vi "New JSON ({Boolean[]}).vi"(7 "keys":string[](array[string]), 8 "error in (no error)":errorcluster, 10 "values":bool[](array[boolean])) -> (0 "error out":errorcluster, 3 "JSON Value out":refnum<class "JSON Value.lvclass">)   [LabVIEW 2016, in "JSON Value.lvclass"]
doc: "Create a new JSON Object initialized with the given key value pairs. The key and value arrays must be the same size."
uses:
  JSON Value.lvclass
  Object/Insert Value/Insert Value (Value[]).vi
  New JSON (Boolean).vi
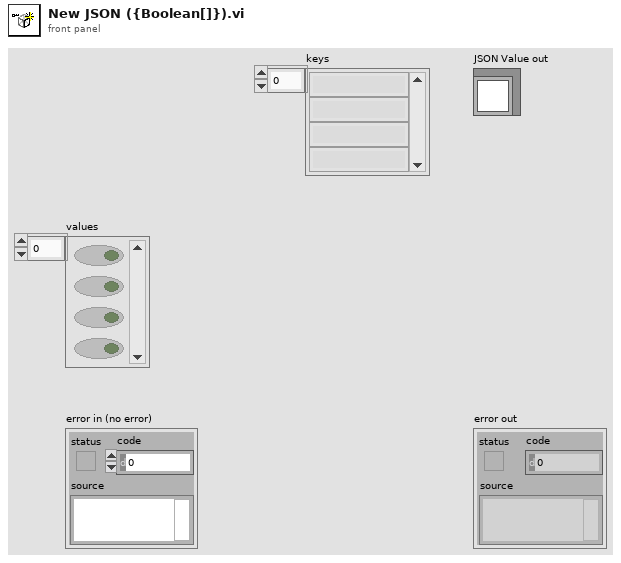
[diagram p1: front panel]
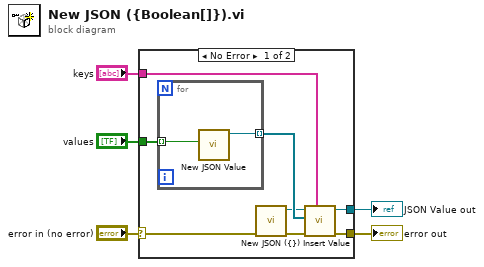
[diagram p0: block diagram]
diagram:
  n1 = case shown="No Error" "error in (no error)" {
    selector: "error in (no error)" -> [w13 w16]
    tunnel: [w12 w16] -> w4
    tunnel: [w11 _] -> w3
    tunnel: "keys" -> [w10 _]
    tunnel: "values" -> [w9 _]
    frame No Error {
      n2 = for {
        tunnel: w9 -> [w15] mode=indexing
        tunnel: [w14] -> w8 mode=indexing
        n3 = call-poly "New JSON Value.vi"("value"=w15) -> ("JSON Value out"=w14:refnum<class "JSON Value.lvclass">)  [unwired: 9 in, 1 out]
      }
      n4 = call "New JSON ({}).vi"("error in (no error)"=w13) -> ("error out"=w7:errorcluster, "JSON Value out"=w6:refnum<class "JSON Value.lvclass">)  [unwired: 9 in]
      n5 = call-poly "Insert Value.vi"("keys"=w10, "error in (no error)"=w7, "values"=w8, "JSON Value in"=w6) -> ("error out"=w12:errorcluster, "JSON Value out"=w11:refnum<class "JSON Value.lvclass">)  [unwired: 5 in, 1 out]
    }
    frame Error {
    }
  }
  "error out" <- w4
  "JSON Value out" <- w3
